vi "contMotionAcq.vi"(0 "sCMOS handle":u32, 1 "fine axial vel (mm/s)":dbl, 2 "coarse axial vel (mm/s)":dbl, 5 "System no.":i32, 7 "zIdx":i32, 9 "z2":dbl, 11 "imgFilenames":path[](array[path]), 12 "stageAccDelay (ms)":u32, 13 "acqDelay (ms)":u32) -> (8 "Controller error":bool)   [LabVIEW 2015]
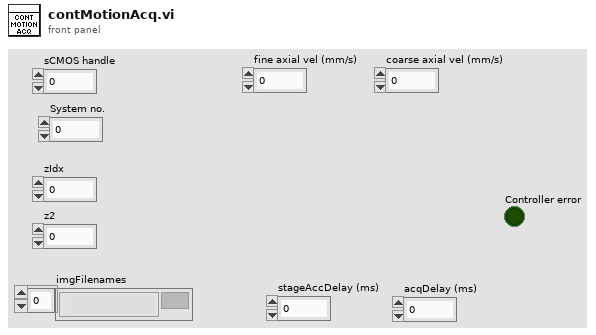
[diagram p1: front panel]
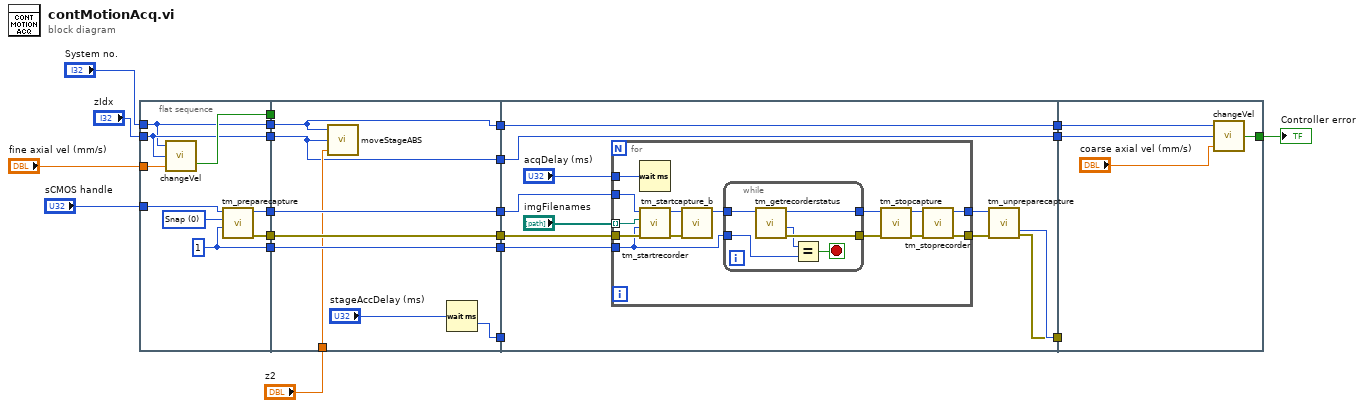
[diagram p0: block diagram]
diagram:
  n1 = flat-sequence {
    tunnel: "fine axial vel (mm/s)" -> [w31]
    tunnel: "zIdx" -> [w24]
    tunnel: "System no." -> [w23]
    tunnel: "sCMOS handle" -> [w28]
    tunnel: [w30] -> w18
    tunnel: [w27] -> w17
    tunnel: [w26] -> w16
    tunnel: [w25] -> w15
    tunnel: [w24] -> w10
    tunnel: [w23] -> w9
    tunnel: w18 -> [_]
    tunnel: w17 -> [w37]
    tunnel: w16 -> [w38]
    tunnel: w15 -> [w39]
    tunnel: [w39] -> w14
    tunnel: [w38] -> w13
    tunnel: [w37] -> w12
    tunnel: "z2" -> [w36]
    tunnel: w10 -> [w32]
    tunnel: w9 -> [w33]
    tunnel: [w34] -> w8
    tunnel: [w33] -> w6
    tunnel: [w32] -> w4
    tunnel: w14 -> [w49]
    tunnel: w13 -> [w48]
    tunnel: w12 -> [w47]
    tunnel: w8 -> [_]
    tunnel: [w45] -> w7
    tunnel: w6 -> [w45]
    tunnel: [w44] -> w5
    tunnel: w4 -> [w44]
    tunnel: [w41] -> w2
    tunnel: [w40] -> w1
    tunnel: w7 -> [w74]
    tunnel: w5 -> [w73]
    tunnel: [w71] -> w3
    tunnel: w2 -> [_]
    tunnel: w1 -> [_]
    frame #0 {
      w27 = 1 ("Frames")
      w29 = 0 items=["Snap", "Sequence"] ("Capture mode")
      n2 = call "changeVel.vi"("vel (mm/s)"=w31, "systemIdx"=w24, "System no."=w23) -> ("Controller error"=w30:bool)
      n3 = call <userlib>:"tm_preparecapture.vi"("Frames"=w27, "Capture mode"=w29, "Handle in"=w28) -> ("error out"=w26:errorcluster, "Handle out"=w25:u32)  [unwired: 5 in, 2 out]
    }
    frame #1 {
      n4 = call "moveStageABS.vi"("absolute pos (mm)"=w36, "axisIdx"=w32, "System no."=w33) -> ()  [unwired: 1 out]
      n5 = Wait (ms)(milliseconds to wait="stageAccDelay (ms)") -> (millisecond timer value=w34:u32)
    }
    frame #2 {
      n6 = for {
        tunnel: w49 -> [w63]
        tunnel: [w58] -> w43
        tunnel: w48 -> [w64]
        tunnel: [w57] -> w42
        tunnel: w47 -> [w51]
        tunnel: "imgFilenames" -> [w56] mode=indexing
        tunnel: "acqDelay (ms)" -> [w55]
        n7 = Wait (ms)(milliseconds to wait=w55) -> ()  [unwired: 1 out]
        n8 = call <userlib>:"tm_startrecorder.vi"("error in (no error)"=w64, "frames"=w51, "File"=w56, "Handle in"=w63) -> ("error out"=w61:errorcluster, "Handle out"=w62:u32)  [unwired: 6 in]
        n9 = call <userlib>:"tm_startcapture_b.vi"("error in (no error)"=w61, "Handle in"=w62) -> ("Handle out"=w54:u32)  [unwired: 8 in, 1 out]
        n10 = while {
          tunnel: w54 -> [w70]
          tunnel: [w69] -> w53
          tunnel: [w68] -> w52
          tunnel: w51 -> [w65]
          stop <- w67 stop-if-true
          n11 = call <userlib>:"tm_getrecorderstatus.vi"("Handle"=w70) -> ("error out"=w68:errorcluster, "Count"=w66:i32, "Handle"=w69:u32)  [unwired: 7 in, 1 out]
          n12 = Equal?(x=w66, y=w65) -> (x = y?=w67:bool)
        }
        n13 = call <userlib>:"tm_stopcapture.vi"("error in (no error)"=w52, "Handle in"=w53) -> ("error out"=w59:errorcluster, "Handle out"=w60:u32)  [unwired: 8 in]
        n14 = call <userlib>:"tm_stoprecorder.vi"("error in (no error)"=w59, "Handle in"=w60) -> ("error out"=w57:errorcluster, "Handle out"=w58:u32)  [unwired: 8 in]
      }
      n15 = call <userlib>:"tm_unpreparecapture.vi"("error in (no error)"=w42, "Handle in"=w43) -> ("error out"=w40:errorcluster, "Handle out"=w41:u32)  [unwired: 8 in]
    }
    frame #3 {
      n16 = call "changeVel.vi"("vel (mm/s)"="coarse axial vel (mm/s)", "systemIdx"=w73, "System no."=w74) -> ("Controller error"=w71:bool)
    }
  }
  "Controller error" <- w3
